vi "Timer Data.vi"(8 "error in (no error)":errorcluster, 11 "LV Server in":refnum<class "LV Server.lvclass">) -> (0 "error out":errorcluster, 1 "Timer Value":string, 2 "Timer State":string, 3 "LV Server out":refnum<class "LV Server.lvclass">)   [LabVIEW 2020, in "LV Server.lvclass"]
uses:
  LV Server.lvclass
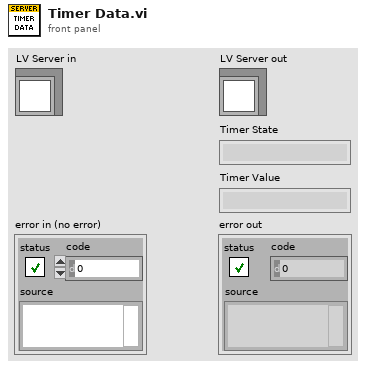
[diagram p1: front panel]
types:
  T1 = typedef "LV Server.lvclass/Timer Data.ctl" = cluster{"Start":dbl, "Accumulated":dbl, "Running":bool}
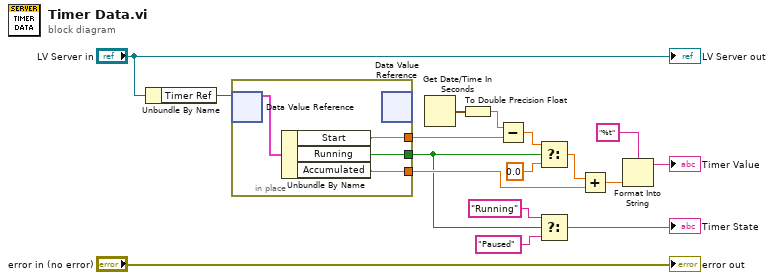
[diagram p0: block diagram]
diagram:
  n1 = Unbundle By Name("LV Server in") -> ("Timer Ref"=w16:refnum<data-value>)
  n2 = in-place {
    in-place-border: [w20] -> w13
    in-place-border: [w19] -> w7
    in-place-border: [w18] -> w9
    n3 = in-place-dvr #1(w16) -> (w21:T1)  [unwired: 1 out]
    n4 = Unbundle By Name(w21) -> ("Start"=w20:dbl, "Running"=w19:bool, "Accumulated"=w18:dbl)
    n5 = in-place-dvr #1() -> ()  [unwired: 1 in, 2 out]
  }
  n6 = Get Date/Time In Seconds() -> (seconds since 1Jan1904=w14:timestamp)
  n7 = To Double Precision Float(number=w14) -> (double precision float=w12:dbl)
  n8 = Subtract(x=w12, y=w13) -> (x-y=w11:dbl)
  n9 = Select(t=w11, s=w7, f=0.0) -> (s? t:f=w8:dbl)
  n10 = Select(t="Running", s=w7, f="Paused") -> (s? t:f=→"Timer State":string)
  n11 = Add(x=w8, y=w9) -> (x+y=w3:dbl)
  n12 = Format Into String(format string="%t", w3) -> (resulting string=→"Timer Value":string)  [unwired: 2 in, 1 out]
  "error out" <- "error in (no error)"
  "LV Server out" <- "LV Server in"
